vi "Looper.vi"(8 "error in (no error)":errorcluster, 11 "RSA in":refnum<class "RSA.lvclass">) -> (0 "error out":errorcluster, 3 "RSA out":refnum<class "RSA.lvclass">)   [LabVIEW 2012, in "RSA.lvclass"]
uses:
  RSA.lvclass
  <vilib>/Distrio/Murmex/GenericMessage/GenericMessage.lvclass
  RSA.lvclass/RSA.ctl
  <vilib>/Distrio/Murmex/ResetMessage/ResetMessage.lvclass
  <vilib>/Distrio/Murmex/StopMessage/StopMessage.lvclass
  <vilib>/Distrio/Murmex/Message/Add or replace parameter.vi
  <vilib>/Distrio/Murmex/Murmex/Murmex.lvclass
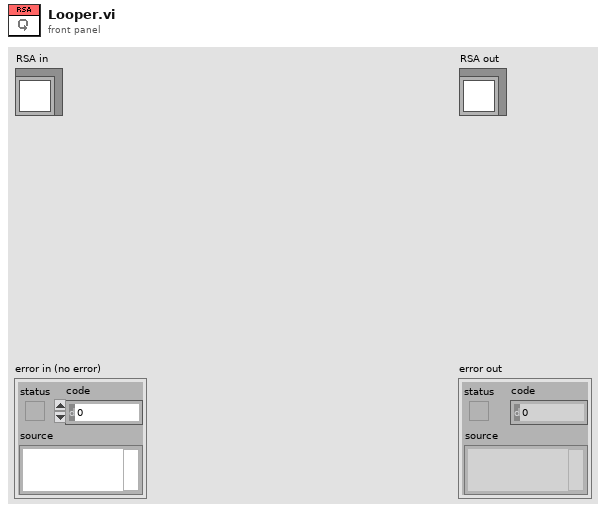
[diagram p1: front panel]
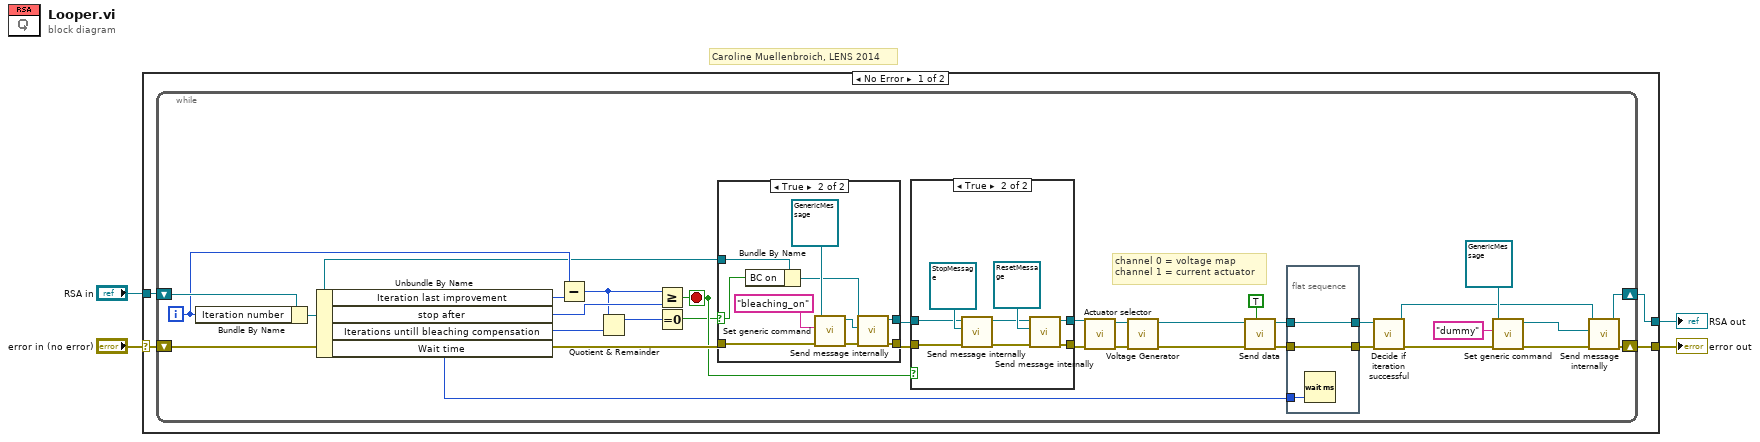
[diagram p0: block diagram]
diagram:
  # "Caroline Muellenbroich, LENS 2014"
  n1 = case shown="No Error" "error in (no error)" {
    selector: "error in (no error)" -> [w7 w68]
    tunnel: [w5 w68] -> w3
    tunnel: [w6 w67] -> w1
    tunnel: "RSA in" -> [w8 w67]
    frame No Error {
      n2 = while {
        shift-right: [w16] -> w6
        shift-left: w8 -> [w41]
        shift-right: [w15] -> w5
        shift-left: w7 -> [w37]
        i -> [w40]
        stop <- w33 stop-if-true
        # "channel 0 = voltage map\nchannel 1 = current actuator"
        n3 = Bundle By Name(cluster=w41, "Iteration number"=w40) -> (w38:refnum<class "RSA.lvclass">)
        n4 = Unbundle By Name(w38) -> ("Iteration last improvement"=w34:i32, "stop after"=w39:i32, "Iterations untill bleaching compensation"=w22:i32, "Wait time"=w24:u32)
        n5 = Subtract(x=w40, y=w34) -> (x-y=w23:i32)
        n6 = Quotient & Remainder(x=w23, y=w22) -> (x-y*floor(x/y)=w21:i32)  [unwired: 1 out]
        n7 = Greater Or Equal?(x=w23, y=w39) -> (x >= y?=w33:bool)
        n8 = Equal To 0?(x=w21) -> (x = 0?=w18:bool)
        n9 = case shown="True" w18 {
          selector: w18 -> [_ w47]
          tunnel: w38 -> [w46 w50]
          tunnel: [w46 w52] -> w35
          tunnel: w37 -> [w45 w53]
          tunnel: [w45 w51] -> w36
          frame False {
          }
          frame True {
            n10 = Bundle By Name(cluster=w50, "BC on"=w47) -> (w49:refnum<class "RSA.lvclass">)
            n11 = call <vilib>:"Set generic command.vi"("error in (no error)"=w53, "generic command"="bleaching_on", "GenericMessage in"=refnum<class "GenericMessage.lvclass"> refnum ("Murmex.lvlib:GenericMessage")) -> ("error out"=w55:errorcluster, "GenericMessage out"=w48:refnum<class "GenericMessage.lvclass">)  [unwired: 7 in]
            n12 = call <vilib>:"Send message internally.vi"("error in (no error)"=w55, "Message"=w48, "Murmex in"=w49) -> ("error out"=w51:errorcluster, "Murmex out"=w52:refnum<class "RSA.lvclass">)  [unwired: 7 in]
          }
        }
        n13 = case shown="True" w33 {
          tunnel: w36 -> [w57 w63]
          tunnel: w35 -> [w58 w60]
          tunnel: [w58 w66] -> w17
          tunnel: [w57 w65] -> w32
          frame False {
          }
          frame True {
            n14 = call <vilib>:"Send message internally.vi"("error in (no error)"=w63, "Message"=refnum<class "StopMessage.lvclass"> refnum ("Murmex.lvlib:StopMessage"), "Murmex in"=w60) -> ("error out"=w62:errorcluster, "Murmex out"=w59:refnum<class "RSA.lvclass">)  [unwired: 7 in]
            n15 = call <vilib>:"Send message internally.vi"("error in (no error)"=w62, "Message"=refnum<class "ResetMessage.lvclass"> refnum ("Message in"), "Murmex in"=w59) -> ("error out"=w65:errorcluster, "Murmex out"=w66:refnum<class "RSA.lvclass">)  [unwired: 7 in]
          }
        }
        n16 = call-dynamic "Actuator selector.vi"("error in (no error)"=w32, "RSA in"=w17) -> ("error out"=w19:errorcluster, "RSA out"=w20:refnum<class "RSA.lvclass">)  [unwired: 8 in]
        n17 = call "Voltage Generator.vi"("error in (no error)"=w19, "RSA in"=w20) -> ("error out"=w30:errorcluster, "RSA out"=w31:refnum<class "RSA.lvclass">)  [unwired: 8 in]
        n18 = call <vilib>:"Send data.vi"("is finalised data? (T)"=TRUE, "error in (no error)"=w30, "Murmex in"=w31) -> ("error out"=w28:errorcluster, "Murmex out"=w26:refnum<class "RSA.lvclass">)  [unwired: 7 in]
        n19 = flat-sequence {
          tunnel: w28 -> [w44]
          tunnel: [w44] -> w27
          tunnel: w26 -> [w43]
          tunnel: [w43] -> w25
          tunnel: w24 -> [w42]
          frame #0 {
            n20 = Wait (ms)(milliseconds to wait=w42) -> ()  [unwired: 1 out]
          }
        }
        n21 = call-dynamic "Decide if iteration successful.vi"("error in (no error)"=w27, "RSA in"=w25) -> ("error out"=w12:errorcluster, "RSA out"=w9:refnum<class "RSA.lvclass">)  [unwired: 8 in]
        n22 = call <vilib>:"Set generic command.vi"("error in (no error)"=w12, "generic command"="dummy", "GenericMessage in"=refnum<class "GenericMessage.lvclass"> refnum ("Murmex.lvlib:GenericMessage")) -> ("error out"=w11:errorcluster, "GenericMessage out"=w10:refnum<class "GenericMessage.lvclass">)  [unwired: 7 in]
        n23 = call <vilib>:"Send message internally.vi"("error in (no error)"=w11, "Message"=w10, "Murmex in"=w9) -> ("error out"=w15:errorcluster, "Murmex out"=w16:refnum<class "RSA.lvclass">)  [unwired: 7 in]
      }
    }
    frame Error {
    }
  }
  "error out" <- w3
  "RSA out" <- w1
